vi "Generate waveform.vi"(8 "error in (no error)":errorcluster, 11 "Galvo in":refnum<class "ImagingModeSPIM.lvclass">) -> (0 "error out":errorcluster, 2 "Array":variant[](array[variant]), 3 "Galvo out":refnum<class "ImagingModeSPIM.lvclass">)   [LabVIEW 2012, in "ImagingModeSPIM.lvclass"]
uses:
  ImagingModeSPIM.lvclass
  ImagingModeSPIM.lvclass/ImagingModeSPIM.ctl
  <vilib>/measure/NI_MABase.lvlib
panel:
  out "Mixed Signal Graph":T1(graph)
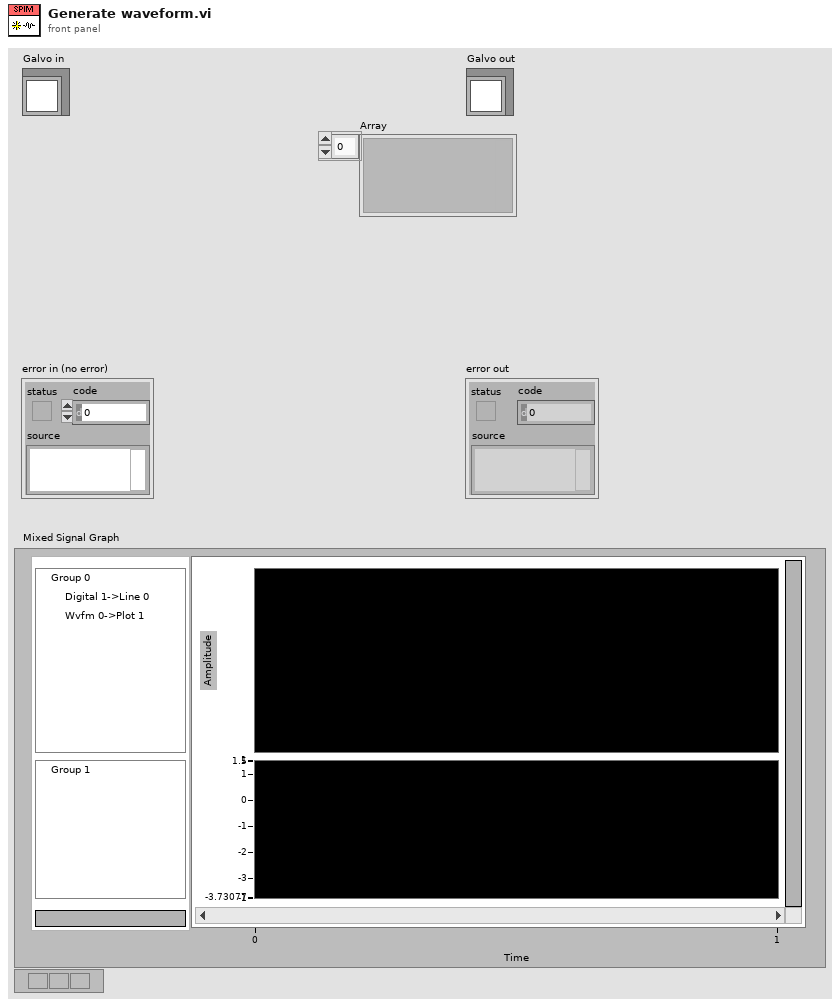
[diagram p1: front panel]
types:
  T1 = cluster{waveform(dbl)[], "digital waveform out":digitalwaveform}
  T2 = typedef "ImagingModeSPIM.lvclass/waveform_enum.ctl" = enum16{"triangular", "sawtooth", "sinusodial"}
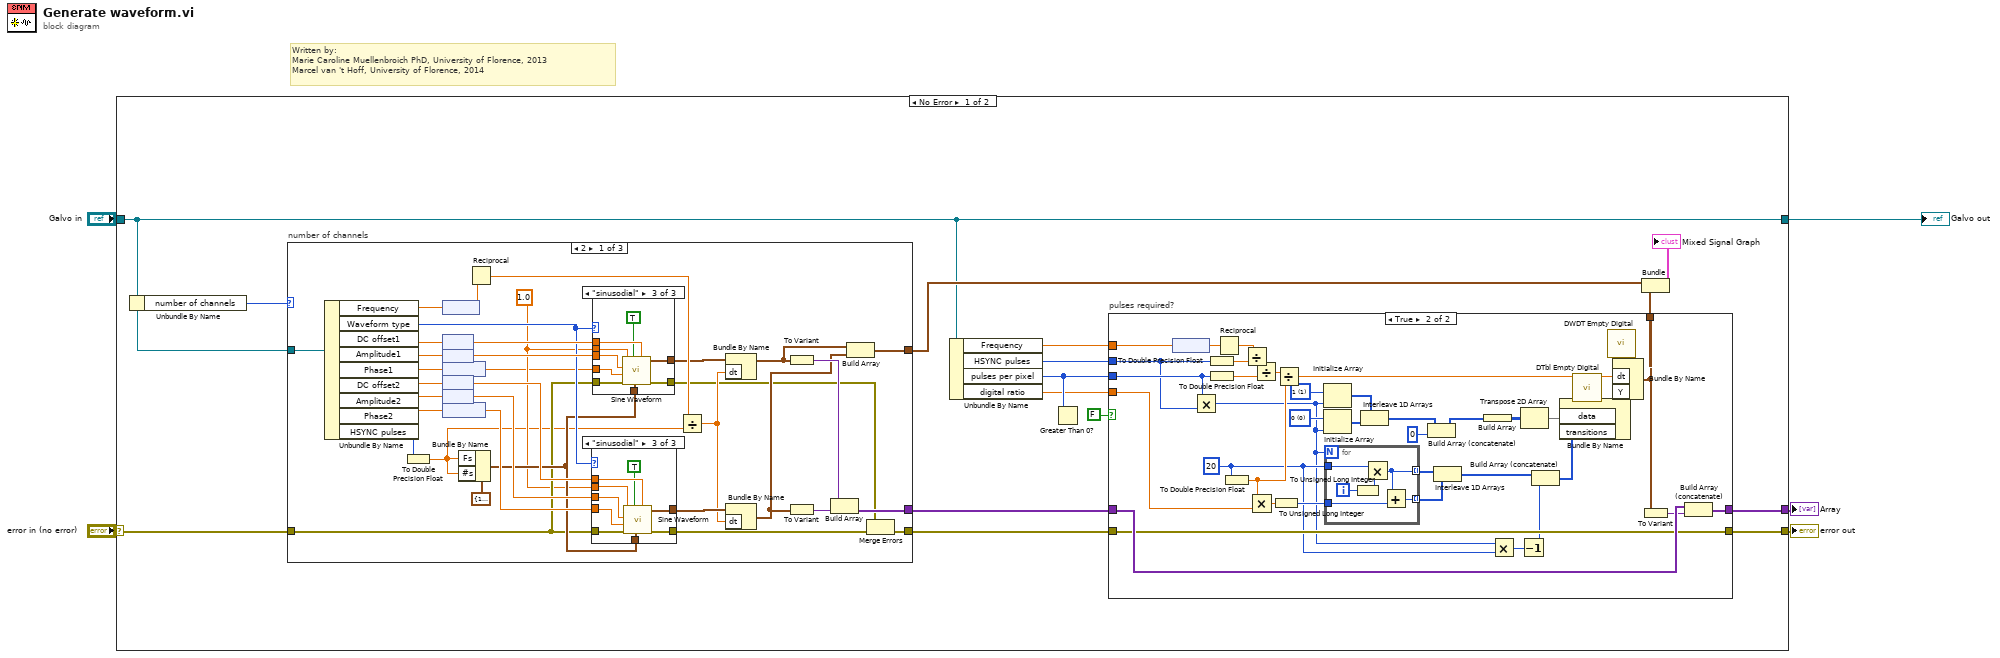
[diagram p0: block diagram]
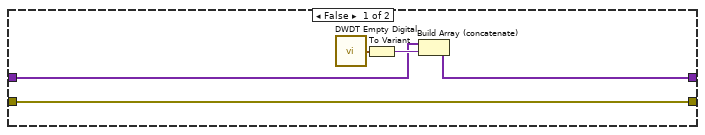
[diagram p2: hidden frame]
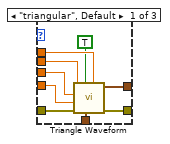
[diagram p3: hidden frame]
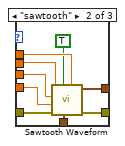
[diagram p4: hidden frame]
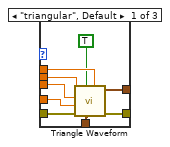
[diagram p5: hidden frame]
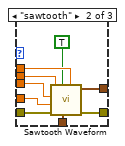
[diagram p6: hidden frame]
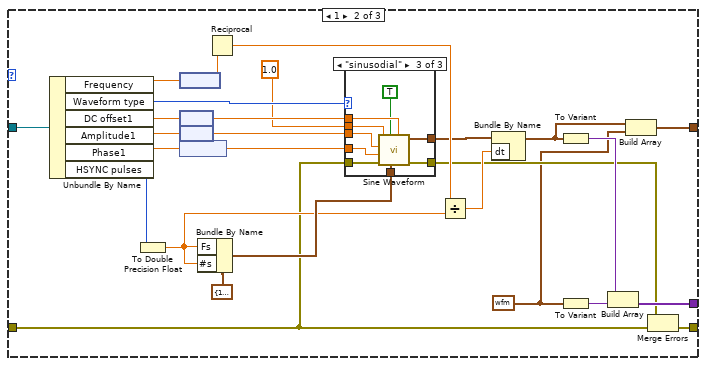
[diagram p7: hidden frame]
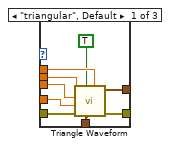
[diagram p8: hidden frame]
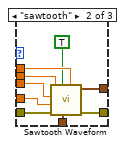
[diagram p9: hidden frame]
diagram:
  # "Written by:\nMarie Caroline Muellenbroich PhD, University of Florence, 2013 \nMarcel van 't Hoff, University of Florence, 2014"
  n1 = case shown="No Error" "error in (no error)" {
    selector: "error in (no error)" -> [w20 w216]
    tunnel: [w12 w216] -> w5
    tunnel: [w8 w215] -> w4
    tunnel: "Galvo in" -> [w8 w215]
    tunnel: [w18 _] -> w3
    frame No Error {
      n2 = Unbundle By Name(w8) -> ("number of channels"=w6:u8)
      n3 = case "number of channels" shown="2" w6 {
        tunnel: [w89 w177 w214] -> w19
        tunnel: w20 -> [w90 w162 w214]
        tunnel: [w88 w176 _] -> w17
        tunnel: [w74 w165 _] -> w10
        tunnel: w8 -> [w71 w160 _]
        frame 2 {
          w84 = 1.0
          n4 = Unbundle By Name(w71) -> ("Frequency"=w81:dbl[unit], "Waveform type"=w99:T2, "DC offset1"=w100:dbl[unit], "Amplitude1"=w101:dbl[unit], "Phase1"=w102:dbl[unit], "DC offset2"=w97:dbl[unit], "Amplitude2"=w96:dbl[unit], "Phase2"=w95:dbl[unit], "HSYNC pulses"=w94:i32)
          n5 = To Double Precision Float(number=w94) -> (double precision float=w79:dbl)
          n6 = node(w81) -> (w83:dbl)
          n7 = node(w100) -> (w104:dbl)
          n8 = node(w101) -> (w105:dbl)
          n9 = node(w102) -> (w80:dbl)
          n10 = node(w97) -> (w98:dbl)
          n11 = node(w96) -> (w92:dbl)
          n12 = node(w95) -> (w93:dbl)
          n13 = Bundle By Name(cluster=cluster{"Fs":dbl, "#s":dbl} {"Fs"=1000.0, "#s"=1000.0} ("sampling info"), "Fs"=w79, "#s"=w79) -> (w91:cluster{"Fs":dbl, "#s":dbl})
          n14 = Reciprocal(x=w83) -> (1/x=w78:dbl)
          n15 = case shown="\"sinusodial\"" w99 {
            tunnel: w98 -> [w112 w123 w132]
            tunnel: w84 -> [w111 w122 w131]
            tunnel: w91 -> [w113 w121 w130]
            tunnel: [w110 w120 w129] -> w82
            tunnel: [w114 w115 w124] -> w85
            tunnel: w92 -> [w107 w118 w127]
            tunnel: w93 -> [w108 w117 w126]
            tunnel: w90 -> [w106 w116 w125]
            frame "triangular", Default {
              n16 = call <vilib>:"Triangle Waveform.vi"("offset"=w112, "sampling info"=w113, "reset signal"=TRUE, "error in (no error)"=w106, "phase"=w108, "amplitude"=w107, "frequency"=w111) -> ("error out"=w114:errorcluster, "signal out"=w110:waveform(dbl))  [unwired: 3 in]
            }
            frame "sawtooth" {
              n17 = call <vilib>:"Sawtooth Waveform.vi"("offset"=w123, "sampling info"=w121, "reset signal"=TRUE, "error in (no error)"=w116, "phase"=w117, "amplitude"=w118, "frequency"=w122) -> ("error out"=w115:errorcluster, "signal out"=w120:waveform(dbl))  [unwired: 3 in]
            }
            frame "sinusodial" {
              n18 = call <vilib>:"Sine Waveform.vi"("offset"=w132, "sampling info"=w130, "reset signal"=TRUE, "error in (no error)"=w125, "phase"=w126, "amplitude"=w127, "frequency"=w131) -> ("error out"=w124:errorcluster, "signal out"=w129:waveform(dbl))  [unwired: 3 in]
            }
          }
          n19 = case shown="\"sinusodial\"" w99 {
            tunnel: w104 -> [w139 w150 w159]
            tunnel: w84 -> [w138 w149 w158]
            tunnel: w105 -> [w137 w148 w157]
            tunnel: w80 -> [w136 w147 w156]
            tunnel: w91 -> [w140 w146 w155]
            tunnel: [w135 w145 w154] -> w75
            tunnel: [w141 w144 w153] -> w72
            tunnel: w90 -> [w133 w142 w151]
            frame "triangular", Default {
              n20 = call <vilib>:"Triangle Waveform.vi"("offset"=w139, "sampling info"=w140, "reset signal"=TRUE, "error in (no error)"=w133, "phase"=w136, "amplitude"=w137, "frequency"=w138) -> ("error out"=w141:errorcluster, "signal out"=w135:waveform(dbl))  [unwired: 3 in]
            }
            frame "sawtooth" {
              n21 = call <vilib>:"Sawtooth Waveform.vi"("offset"=w150, "sampling info"=w146, "reset signal"=TRUE, "error in (no error)"=w142, "phase"=w147, "amplitude"=w148, "frequency"=w149) -> ("error out"=w144:errorcluster, "signal out"=w145:waveform(dbl))  [unwired: 3 in]
            }
            frame "sinusodial" {
              n22 = call <vilib>:"Sine Waveform.vi"("offset"=w159, "sampling info"=w155, "reset signal"=TRUE, "error in (no error)"=w151, "phase"=w156, "amplitude"=w157, "frequency"=w158) -> ("error out"=w153:errorcluster, "signal out"=w154:waveform(dbl))  [unwired: 3 in]
            }
          }
          n23 = Divide(x=w78, y=w79) -> (x/y=w77:dbl)
          n24 = Bundle By Name(cluster=w75, "dt"=w77) -> (w73:waveform(dbl))
          n25 = Bundle By Name(cluster=w82, "dt"=w77) -> (w76:waveform(dbl))
          n26 = To Variant(anything=w73) -> (Variant=w86:variant)
          n27 = To Variant(anything=w76) -> (Variant=w87:variant)
          n28 = Build Array(w86, w87) -> (w88:variant[])
          n29 = Build Array(w73, w76) -> (w74:waveform(dbl)[])
          n30 = Merge Errors(w72, w85) -> (w89:errorcluster)
        }
        frame 1 {
          w161 = waveform(dbl) {"t0"=timestamp(0 s since 1904-01-01), "dt"=1.0, "Y"=[]} ("signal out")
          n31 = Unbundle By Name(w160) -> ("Frequency"=w171:dbl[unit], "Waveform type"=w180:T2, "DC offset1"=w181:dbl[unit], "Amplitude1"=w182:dbl[unit], "Phase1"=w183:dbl[unit], "HSYNC pulses"=w179:i32)
          n32 = To Double Precision Float(number=w179) -> (double precision float=w169:dbl)
          n33 = node(w171) -> (w172:dbl)
          n34 = node(w181) -> (w185:dbl)
          n35 = node(w182) -> (w186:dbl)
          n36 = node(w183) -> (w170:dbl)
          n37 = Bundle By Name(cluster=cluster{"Fs":dbl, "#s":dbl} {"Fs"=1000.0, "#s"=1000.0} ("sampling info"), "Fs"=w169, "#s"=w169) -> (w178:cluster{"Fs":dbl, "#s":dbl})
          n38 = Reciprocal(x=w172) -> (1/x=w168:dbl)
          n39 = case shown="\"sinusodial\"" w180 {
            tunnel: w185 -> [w193 w204 w213]
            tunnel: 1.0 -> [w192 w203 w212]
            tunnel: w186 -> [w191 w202 w211]
            tunnel: w170 -> [w190 w201 w210]
            tunnel: w178 -> [w194 w200 w209]
            tunnel: [w189 w199 w208] -> w166
            tunnel: [w195 w198 w207] -> w163
            tunnel: w162 -> [w187 w196 w205]
            frame "triangular", Default {
              n40 = call <vilib>:"Triangle Waveform.vi"("offset"=w193, "sampling info"=w194, "reset signal"=TRUE, "error in (no error)"=w187, "phase"=w190, "amplitude"=w191, "frequency"=w192) -> ("error out"=w195:errorcluster, "signal out"=w189:waveform(dbl))  [unwired: 3 in]
            }
            frame "sawtooth" {
              n41 = call <vilib>:"Sawtooth Waveform.vi"("offset"=w204, "sampling info"=w200, "reset signal"=TRUE, "error in (no error)"=w196, "phase"=w201, "amplitude"=w202, "frequency"=w203) -> ("error out"=w198:errorcluster, "signal out"=w199:waveform(dbl))  [unwired: 3 in]
            }
            frame "sinusodial" {
              n42 = call <vilib>:"Sine Waveform.vi"("offset"=w213, "sampling info"=w209, "reset signal"=TRUE, "error in (no error)"=w205, "phase"=w210, "amplitude"=w211, "frequency"=w212) -> ("error out"=w207:errorcluster, "signal out"=w208:waveform(dbl))  [unwired: 3 in]
            }
          }
          n43 = Divide(x=w168, y=w169) -> (x/y=w167:dbl)
          n44 = Bundle By Name(cluster=w166, "dt"=w167) -> (w164:waveform(dbl))
          n45 = To Variant(anything=w164) -> (Variant=w174:variant)
          n46 = To Variant(anything=w161) -> (Variant=w175:variant)
          n47 = Build Array(w174, w175) -> (w176:variant[])
          n48 = Build Array(w164, w161) -> (w165:waveform(dbl)[])
          n49 = Merge Errors(w163, w162) -> (w177:errorcluster)
        }
        frame Default {
        }
      }
      n50 = Unbundle By Name(w8) -> ("Frequency"=w16:dbl[unit], "HSYNC pulses"=w15:i32, "pulses per pixel"=w13:i32, "digital ratio"=w11:dbl)
      n51 = Greater Than 0?(x=w13) -> ()  [unwired: 1 out]
      n52 = case "pulses required?" shown="True" FALSE {
        tunnel: w13 -> [_ w29]
        tunnel: [w25 w46] -> w12
        tunnel: w19 -> [w25 w46]
        tunnel: [w21 w59] -> w18
        tunnel: w17 -> [w22 w60]
        tunnel: w16 -> [_ w64]
        tunnel: w15 -> [_ w26]
        tunnel: [_ w56] -> w9
        tunnel: w11 -> [_ w42]
        frame False {
          n53 = call <vilib>:"DWDT Empty Digital.vi"() -> ("digital waveform out"=w23:digitalwaveform)  [unwired: 5 in]
          n54 = To Variant(anything=w23) -> (Variant=w24:variant)
          n55 = Build Array (concatenate)(w22, w24) -> (w21:variant[])
        }
        frame True {
          w30 = u32 20 ("ratio step size")
          w48 = u8 0 items=["0", "1", "Z", "L", "H", "X", "T", "V"] ("value 2")
          w47 = u8 1 items=["0", "1", "Z", "L", "H", "X", "T", "V"] ("value 2")
          n56 = node(w64) -> (w63:dbl)
          n57 = Multiply(x=w29, y=w26) -> (x*y=w27:i32)
          n58 = To Double Precision Float(number=w26) -> (double precision float=w61:dbl)
          n59 = To Double Precision Float(number=w29) -> (double precision float=w57:dbl)
          n60 = Reciprocal(x=w63) -> (1/x=w62:dbl)
          n61 = To Double Precision Float(number=w30) -> (double precision float=w41:dbl)
          n62 = Divide(x=w62, y=w61) -> (x/y=w58:dbl)
          n63 = Multiply(x=w41, y=w42) -> (x*y=w52:dbl)
          n64 = Divide(x=w58, y=w57) -> (x/y=w40:dbl)
          n65 = To Unsigned Long Integer(number=w52) -> (unsigned 32bit integer=w55:u32)
          n66 = Divide(x=w40, y=w41) -> (x/y=w39:dbl)
          n67 = Initialize Array(w47, w27) -> (w50:u8[])
          n68 = Initialize Array(w48, w27) -> (w51:u8[])
          n69 = for {
            N: w27 -> [_]
            tunnel: w55 -> [w68]
            tunnel: w30 -> [w70]
            tunnel: [w67] -> w53 mode=indexing
            tunnel: [w66] -> w54 mode=indexing
            i -> [w69]
            n70 = To Unsigned Long Integer(number=w69) -> (unsigned 32bit integer=w65:u32)
            n71 = Multiply(x=w70, y=w65) -> (x*y=w67:u32)
            n72 = Add(x=w67, y=w68) -> (x+y=w66:u32)
          }
          n73 = Interleave 1D Arrays(w50, w51) -> (w35:u8[])
          n74 = Build Array (concatenate)(w35, u8 0 ("value 2")) -> (w34:u8[])
          n75 = Interleave 1D Arrays(w53, w54) -> (w33:u32[])
          n76 = Build Array(w34) -> (w49:u8[][])
          n77 = Multiply(x=w27, y=w30) -> (x*y=w31:u32)
          n78 = Decrement(x=w31) -> (x-1=w28:u32)
          n79 = Transpose 2D Array(2D array=w49) -> (transposed array=w37:u8[][])
          n80 = Build Array (concatenate)(w33, w28) -> (w32:u32[])
          n81 = call <vilib>:"DTbl Empty Digital.vi"() -> ("digital data"=w45:digitaldata)  [unwired: 5 in]
          n82 = Bundle By Name(cluster=w45, "data"=w37, "transitions"=w32) -> (w43:digitaldata)
          n83 = call <vilib>:"DWDT Empty Digital.vi"() -> ("digital waveform out"=w44:digitalwaveform)  [unwired: 5 in]
          n84 = Bundle By Name(cluster=w44, "dt"=w39, "Y"=w43) -> (w56:digitalwaveform)
          n85 = To Variant(anything=w56) -> (Variant=w38:variant)
          n86 = Build Array (concatenate)(w60, w38) -> (w59:variant[])
        }
      }
      n87 = Bundle(w10, "digital waveform out"=w9) -> (→"Mixed Signal Graph":T1)  [unwired: 1 in]
    }
    frame Error {
    }
  }
  "error out" <- w5
  "Galvo out" <- w4
  "Array" <- w3
